vi "Golden Section Inner Part.vi"(1 "result":dbl[](array[numeric]) format="%.2f", 4 "accuracy":dbl format="%.2f", 5 "table":i32[][](array[numeric]), 6 "case":bool, 7 "c (start)":dbl format="%.2f", 8 "list of variables":i32[](array[numeric]), 9 "b (start)":dbl format="%.2f", 10 "a (start)":dbl format="%.2f") -> (0 "error":i32, 2 "f(minimum)":dbl format="%.2f", 3 "minimum":dbl format="%.2f")   [LabVIEW 2020, in "NI_Gmath.lvlib"]
uses:
  <vilib>/gmath/NI_Gmath.lvlib
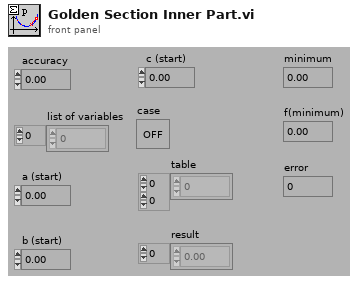
[diagram p1: front panel]
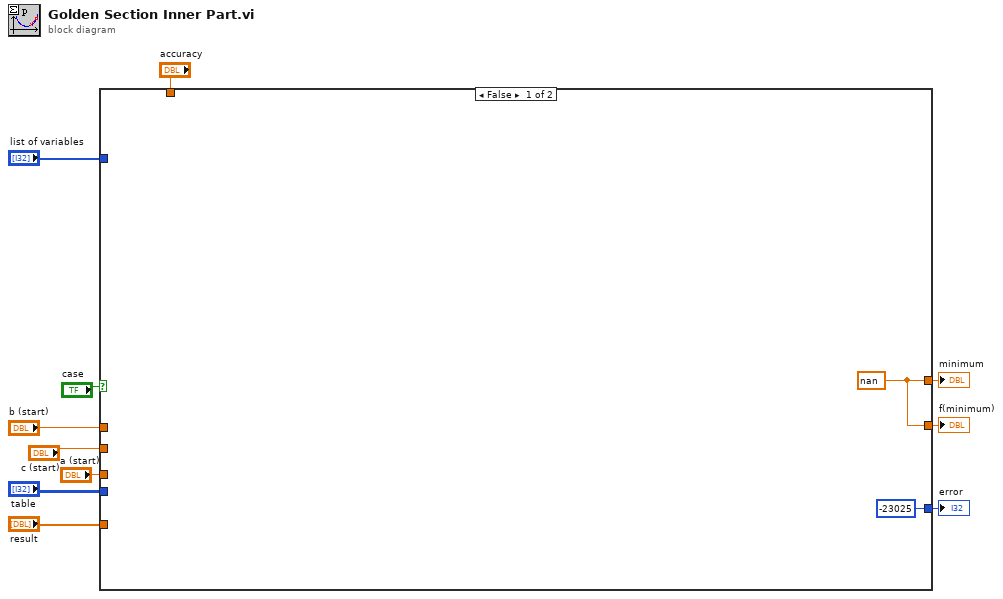
[diagram p0: block diagram]
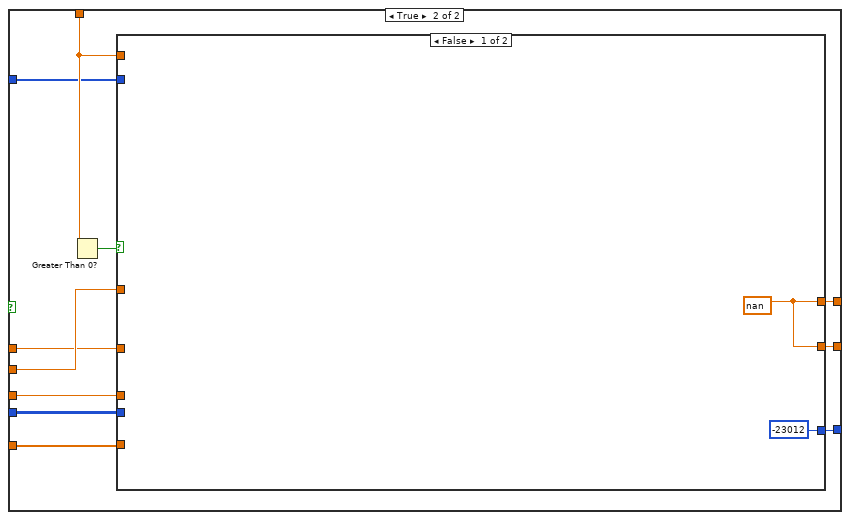
[diagram p2: hidden frame]
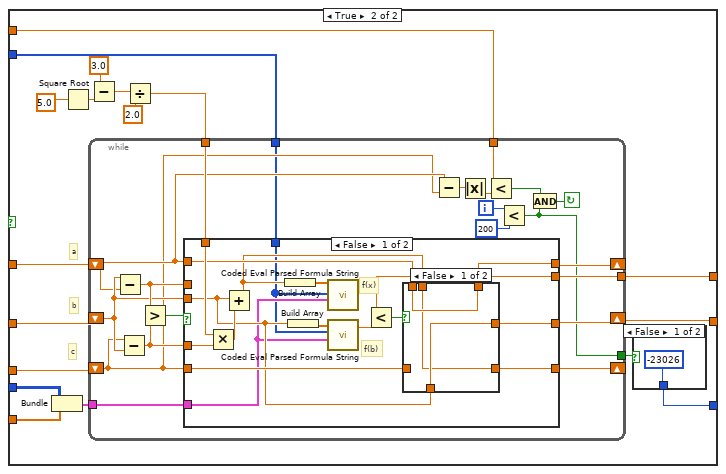
[diagram p3: hidden frame]
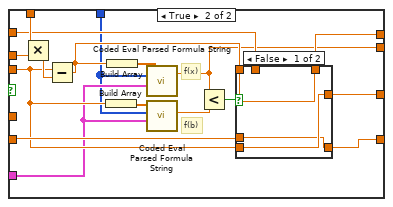
[diagram p5: hidden frame]
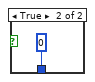
[diagram p7: hidden frame]
diagram:
  n1 = case shown="False" "case" {
    tunnel: "c (start)" -> [_ w24]
    tunnel: "b (start)" -> [_ w23]
    tunnel: "a (start)" -> [_ w22]
    tunnel: [w13 w21] -> w5
    tunnel: [w13 w20] -> w6
    tunnel: [-23025 w18] -> w7
    tunnel: "accuracy" -> [_ w17]
    tunnel: "table" -> [_ w16]
    tunnel: "result" -> [_ w15]
    tunnel: "list of variables" -> [_ w14]
    frame False {
      w13 = nan
    }
    frame True {
      n2 = Greater Than 0?(x=w17) -> (x > 0?=w19:bool)
      n3 = case shown="False" w19 {
        tunnel: [w26 w44] -> w20
        tunnel: [w26 w43] -> w21
        tunnel: w22 -> [_ w42]
        tunnel: w23 -> [_ w41]
        tunnel: w24 -> [_ w40]
        tunnel: w17 -> [_ w33]
        tunnel: [-23012 w31] -> w18
        tunnel: w16 -> [_ w29]
        tunnel: w15 -> [_ w28]
        tunnel: w14 -> [_ w27]
        frame False {
          w26 = nan
        }
        frame True {
          # "a"
          # "b"
          # "c"
          n4 = Bundle("table"=w29, "result"=w28) -> (w30:cluster{"table":i32[][], "result":dbl[]})  [unwired: 1 in]
          n5 = Square Root(x=5.0) -> (sqrt(x)=w36:dbl)
          n6 = Subtract(x=3.0, y=w36) -> (x-y=w37:dbl)
          n7 = Divide(x=w37, y=2.0) -> (x/y=w39:dbl)
          n8 = while {
            tunnel: w27 -> [w45]
            tunnel: w30 -> [w46]
            tunnel: [w47] -> w32
            tunnel: w33 -> [w52]
            tunnel: [w53] -> w43
            tunnel: w39 -> [w64]
            shift-left: w42 -> [w56]
            shift-right: [w60] -> _
            shift-left: w41 -> [w61]
            shift-right: [w54] -> w44
            shift-left: w40 -> [w58]
            shift-right: [w55] -> _
            i -> [w51]
            stop <- w48 continue-if-true
            n9 = Subtract(x=w61, y=w58) -> (x-y=w63:dbl)
            n10 = Subtract(x=w56, y=w61) -> (x-y=w62:dbl)
            n11 = Greater?(x=w63, y=w62) -> (0:w65:bool)
            n12 = case shown="False" w65 {
              tunnel: w61 -> [w71 w95]
              tunnel: w64 -> [w81 w105]
              tunnel: w63 -> [_ w104]
              tunnel: w62 -> [w82 _]
              tunnel: w58 -> [w73 w101]
              tunnel: [w77 w100] -> w55
              tunnel: [w76 w99] -> w54
              tunnel: [w74 w98] -> w60
              tunnel: w56 -> [w75 w97]
              tunnel: [w70 w93] -> w53
              tunnel: w46 -> [w67 w90]
              tunnel: w45 -> [w66 w89]
              frame False {
                # "f(b)"
                # "f(x)"
                n13 = Multiply(x=w81, y=w82) -> (x*y=w80:dbl)
                n14 = Add(x=w71, y=w80) -> (x+y=w72:dbl)
                n15 = Build Array(w72) -> (w68:dbl[])
                n16 = Build Array(w71) -> (w69:dbl[])
                n17 = call <vilib>:"Coded Eval Parsed Formula String.vi"("Parsed Formula"=w67, "Variables"=w66, "X Values"=w68) -> ("y value"=w70:dbl)  [unwired: 1 in, 1 out]
                n18 = call <vilib>:"Coded Eval Parsed Formula String.vi"("Parsed Formula"=w67, "Variables"=w66, "X Values"=w69) -> ("y value"=w79:dbl)  [unwired: 1 in, 1 out]
                n19 = Less?(x=w70, y=w79) -> (x < y?=w78:bool)
                n20 = case shown="False" w78 {
                  tunnel: w71 -> [w84 w88]
                  tunnel: [w85 w88] -> w77
                  tunnel: w72 -> [w83 w87]
                  tunnel: [w84 w87] -> w76
                  tunnel: w75 -> [_ w86]
                  tunnel: [w83 w86] -> w74
                  tunnel: w73 -> [w85 _]
                  frame False {
                  }
                  frame True {
                  }
                }
              }
              frame True {
                # "f(b)"
                # "f(x)"
                n21 = Multiply(x=w105, y=w104) -> (x*y=w103:dbl)
                n22 = Subtract(x=w95, y=w103) -> (x-y=w94:dbl)
                n23 = Build Array(w95) -> (w92:dbl[])
                n24 = Build Array(w94) -> (w91:dbl[])
                n25 = call <vilib>:"Coded Eval Parsed Formula String.vi"("Parsed Formula"=w90, "Variables"=w89, "X Values"=w91) -> ("y value"=w93:dbl)  [unwired: 1 in, 1 out]
                n26 = call <vilib>:"Coded Eval Parsed Formula String.vi"("Parsed Formula"=w90, "Variables"=w89, "X Values"=w92) -> ("y value"=w96:dbl)  [unwired: 1 in, 1 out]
                n27 = Less?(x=w93, y=w96) -> (x < y?=w102:bool)
                n28 = case shown="False" w102 {
                  tunnel: w101 -> [_ w111]
                  tunnel: [w108 w111] -> w100
                  tunnel: w94 -> [w108 w110]
                  tunnel: [w107 w110] -> w99
                  tunnel: w95 -> [w107 w109]
                  tunnel: [w106 w109] -> w98
                  tunnel: w97 -> [w106 _]
                  frame False {
                  }
                  frame True {
                  }
                }
              }
            }
            n29 = Subtract(x=w58, y=w56) -> (x-y=w59:dbl)
            n30 = Absolute Value(x=w59) -> (abs(x)=w57:dbl)
            n31 = Less?(x=w52, y=w57) -> (x < y?=w49:bool)
            n32 = Less?(x=w51, y=200) -> (x < y?=w47:bool)
            n33 = And(x=w49, y=w47) -> (x .and. y?=w48:bool)
          }
          n34 = case shown="False" w32 {
            tunnel: [-23026 0] -> w31
            frame False {
            }
            frame True {
            }
          }
        }
      }
    }
  }
  "error" <- w7
  "f(minimum)" <- w6
  "minimum" <- w5
